vi "Motor_Subsys.vi"(4 "B [Nms]":dbl, 6 "[1/J]":dbl, 7 "Voltage Input [V]":dbl, 9 "K [Nm/Amp]":dbl, 10 "R [ohm]":dbl, 11 "[1/L]":dbl) -> (2 "d_theta":dbl, 3 "theta":dbl)   [LabVIEW 2014]
uses:
  <vilib>/Simulation/Implementation/Shared/SIMSCR Execution Mode.ctl
  <vilib>/Simulation/Scripting/Companion Diagram/SimConfigNode/SimParams.ctl
  <vilib>/Simulation/Scripting/Companion Diagram/SimConfigNode/_simSolvers.ctl
  <vilib>/Simulation/Param Hierarchy/Typedefs/SIMPH Param Control Actions.ctl
  <vilib>/Simulation/Implementation/Shared/SIM limit type.ctl
  <vilib>/Simulation/Implementation/Shared/NILVSim_ParamChanged.vi
  <vilib>/Simulation/Implementation/Shared/NILVSIM_BeginStep.vi
  <vilib>/Simulation/ContinuousLinear/Implementation/NILVSim Integrator new.llb/SIM Integrator distributor (scalar).vi
  <vilib>/Simulation/SignalArithmetic/Implementation/NILVSim Gain.llb/SIM Gain (scalar).vi
  <vilib>/Simulation/ContinuousLinear/Implementation/NILVSim Integrator new.llb/SIM Integrator collector (scalar).vi
  <vilib>/Simulation/Implementation/Shared/NILVSim_Manager.vi
  <vilib>/Utility/error.llb/Clear Errors.vi
  <vilib>/Simulation/Implementation/Shared/NILVSim_FinalizeModel.vi
  <vilib>/Simulation/Implementation/Shared/SIM Unbundle Sim Info.vi
  <vilib>/Simulation/Implementation/Shared/SIMSH Read Queue.vi
  <vilib>/Simulation/Implementation/Shared/NILVSim_Initialize.vi
  <vilib>/Simulation/Utility/Implementation/NILVSim Get Time and IsAcceptedStep.vi
  <vilib>/Simulation/Implementation/Shared/NILVSim_GetModelError.vi
  <vilib>/Simulation/Implementation/Shared/SIM SimErrorHandler.vi
  <vilib>/Simulation/Implementation/Shared/SIM Bundle Sim Info.vi
  <vilib>/Simulation/Scripting/Companion Diagram/SimConfigNode/SimDog.xnode
  <vilib>/Simulation/Implementation/XNodeFramework/SimXNode/SimX.xnode
  <vilib>/Simulation/ContinuousLinear/Implementation/NILVSim Integrator new.llb/SIM Integrator (scalar).vi
  <vilib>/Simulation/Implementation/Shared/NI_SIM_Implementation.lvlib
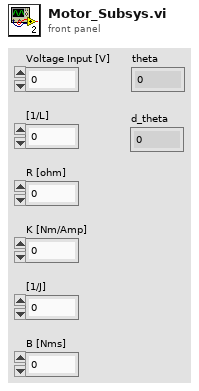
[diagram p1: front panel]
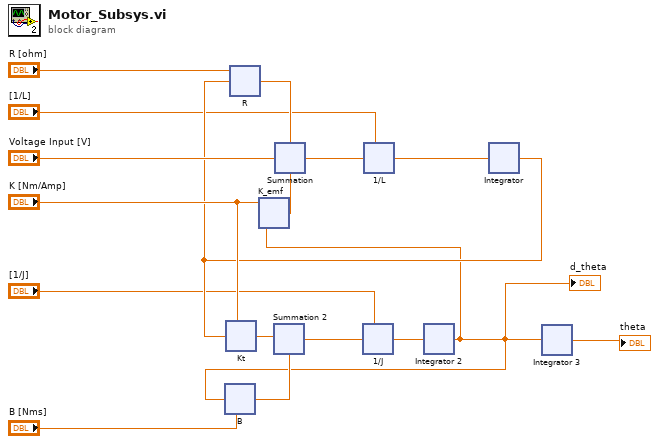
[diagram p0: block diagram]
diagram:
  n1 = xnode "B"("gain"="B [Nms]", "input"=w1) -> ("output"=w9:dbl)  [unwired: 2 in]
  n2 = xnode "Kt"("gain"="K [Nm/Amp]", "input"=w12) -> ("output"=w7:dbl)  [unwired: 2 in]
  n3 = xnode "Summation 2"("Operand1"=w7, "Operand2"=w9) -> ("Result"=w4:dbl)
  n4 = xnode "1/J"("gain"="[1/J]", "input"=w4) -> ("output"=w15:dbl)  [unwired: 2 in]
  n5 = xnode "Integrator 2"("input"=w15) -> ("output"=w1:dbl)  [unwired: 9 in, 2 out]
  "d_theta" <- w1
  n6 = xnode "K_emf"("gain"="K [Nm/Amp]", "input"=w1) -> ("output"=w13:dbl)  [unwired: 2 in]
  n7 = xnode "Integrator 3"("input"=w1) -> ("output"=→"theta":dbl)  [unwired: 9 in, 2 out]
  n8 = xnode "R"("gain"="R [ohm]", "input"=w12) -> ("output"=w11:dbl)  [unwired: 2 in]
  n9 = xnode "Summation"("Operand1"=w11, "Operand2"="Voltage Input [V]", "Operand3"=w13) -> ("Result"=w3:dbl)
  n10 = xnode "1/L"("gain"="[1/L]", "input"=w3) -> ("output"=w2:dbl)  [unwired: 2 in]
  n11 = xnode "Integrator"("input"=w2) -> ("output"=w12:dbl)  [unwired: 9 in, 2 out]
